vi "Set FM Properties.vi"(0 "VISA resource name":refnum<visa-resource-name>, 5 "Channel (0: Channel 1)":T1 items=["Channel 1", "Channel 2"], 7 "FM Source (0: Internal)":u16(ring) items=["Internal", "External"], 9 "Modulation Waveform (0: Sine)":u16(ring) items=["Sine", "Square", "Triangle", "Ramp", "Down Ramp", "Noise", "User 1", "User 2", "User 3", "User 4", "EMEMory", "EFILe"], 11 "error in (no error)":errorcluster, 12 "Modulation Frequency (100.00 Hz)":dbl[unit]=100.0, 13 "Peak Deviation (100.00 Hz)":dbl[unit]=100.0) -> (4 "VISA resource name out":refnum<visa-resource-name>, 15 "error out":errorcluster)   [LabVIEW 2009, in "Tektronix AFG 3000 Series.lvlib"]
uses:
  Tektronix AFG 3000 Series.lvlib
  controls.llb/Channel.ctl
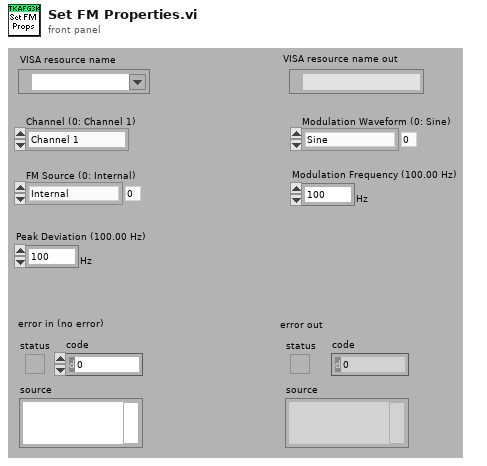
[diagram p1: front panel]
types:
  T1 = typedef "Channel.ctl" = u16
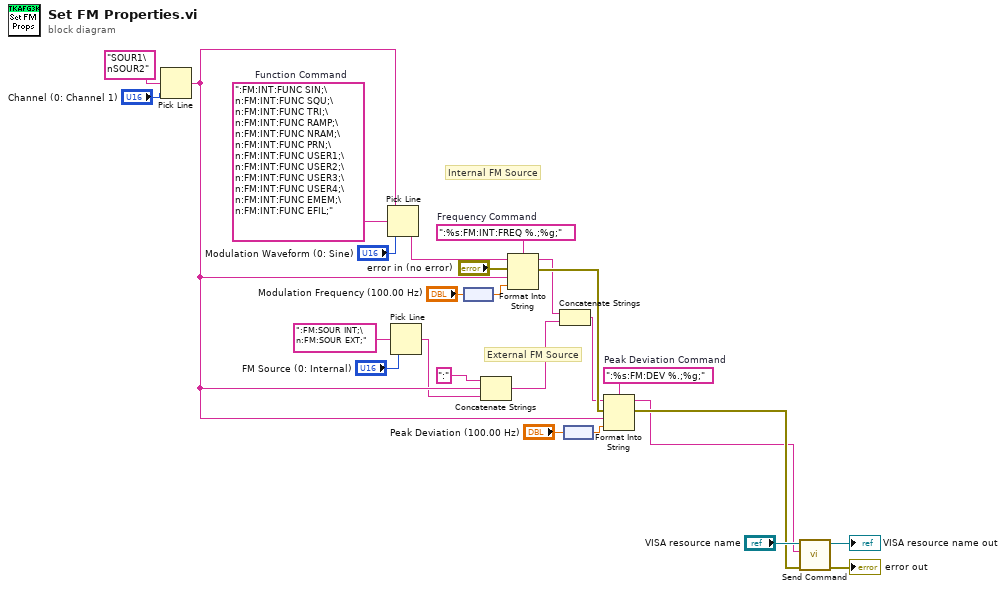
[diagram p0: block diagram]
diagram:
  w18 = ":FM:INT:FUNC SIN;\n:FM:INT:FUNC SQU;\n:FM:INT:FUNC TRI;\n:FM:INT:FUNC RAMP;\n:FM:INT:FUNC NRAM;\n:FM:INT:FUNC PRN;\n:FM:INT:FUNC USER1;\n:FM:INT:FUNC USER2;\n:FM:INT:FUNC USER3;\n:FM:INT:FUNC USER4;\n:FM:INT:FUNC EMEM;\n:FM:INT:FUNC EFIL;"  # Function Command
  w20 = ":%s:FM:INT:FREQ %.;%g;"  # Frequency Command
  w26 = ":%s:FM:DEV %.;%g;"  # Peak Deviation Command
  # "Internal FM Source"
  # "External FM Source"
  n1 = Pick Line(multi-line string="SOUR1\nSOUR2" ("string (\"\")"), line index="Channel (0: Channel 1)") -> (output string=w6:string)  [unwired: 1 out]
  n2 = Pick Line(string ("")=w6, multi-line string=w18, line index="Modulation Waveform (0: Sine)") -> (output string=w19:string)
  n3 = Pick Line(multi-line string=":FM:SOUR INT;\n:FM:SOUR EXT;" ("Source Command"), line index="FM Source (0: Internal)") -> (output string=w5:string)  [unwired: 1 out]
  n4 = node("Modulation Frequency (100.00 Hz)") -> (w14:dbl)
  n5 = Concatenate Strings(":" ("string"), w6, w5) -> (w3:string)
  n6 = Format Into String(format string=w20, initial string=w19, error in="error in (no error)", w6, w14) -> (resulting string=w4:string, error out=w16:errorcluster)
  n7 = Concatenate Strings(w4, w3) -> (w2:string)
  n8 = node("Peak Deviation (100.00 Hz)") -> (w13:dbl)
  n9 = Format Into String(format string=w26, initial string=w2, error in=w16, w6, w13) -> (resulting string=w1:string, error out=w8:errorcluster)
  n10 = call "Send Command.vi"("error in (no error)"=w8, "write buffer"=w1, "VISA resource name"="VISA resource name") -> ("error out"=→"error out":errorcluster, "VISA resource name out"=→"VISA resource name out":refnum<visa-resource-name>)  [unwired: 7 out]
